vi "Read Waveform Measurement.vi"(6 "Source 2 (21: None)":u16(ring)=21 items=["Channel 1", "Channel 2", "Channel 3", "Channel 4", "DIG 0", "DIG 1", "DIG 2", "DIG 3", "DIG 4", "DIG 5", "DIG 6", "DIG 7", "DIG 8", "DIG 9", "DIG 10", "DIG 11", "DIG 12", "DIG 13", "DIG 14", "DIG 15", "Math", "None"], 8 "error in (no error)":errorcluster, 9 "Measurement Function (7: Frequency)":u16(ring)=7 items=["Amplitude", "Voltage Average", "Base", "Counter", "Delay", "Duty Cycle", "Fall Time", "Frequency", "Voltage Max", "Voltage Min", "Overshoot", "Voltage Vpp", "Period", "Phase", "Preshoot", "Rise Time", "Voltage RMS", "Top", "Width Positive", "X at Max Y", "X at Min Y"], 10 "Source 1 (0: Channel 1)":u16(ring) items=["Channel 1", "Channel 2", "Channel 3", "Channel 4", "DIG 0", "DIG 1", "DIG 2", "DIG 3", "DIG 4", "DIG 5", "DIG 6", "DIG 7", "DIG 8", "DIG 9", "DIG 10", "DIG 11", "DIG 12", "DIG 13", "DIG 14", "DIG 15", "Math"], 11 "VISA resource name":refnum<visa-resource-name>="GPIB0::1::INSTR") -> (0 "error out":errorcluster, 2 "Measured Value":dbl, 3 "VISA resource name out":refnum<visa-resource-name>)   [LabVIEW 2021, in "Agilent 6000 Series.lvlib"]
doc: "This VI initiates an acquisition on the channels that you enable with the ag6000a Configure Channel.vi. It then waits for the acquisition to complete, obtains a waveform measurement on the channel you specify, and returns the measurement value. You specify a particular measurement type, such as rise time, frequency, and voltage peak-to-peak. You can call the ag6000a Fetch Waveform Measurement.vi separately for any other waveform measurement that you want to obtain on a specific channel without initiating another acquisition.\n\nNotes:\n(1) You must configure the appropriate reference levels before you call this VI to take a rise time, fall time, width negative, width positive, duty cycle negative, or duty cycle positive measurement.\n(2) You configure the low, mid, and high references either by calling the ag6000a Configure Reference Levels.vi."
uses:
  Agilent 6000 Series.lvlib
  Low Data VIs/Fetch Waveform Measurement.vi
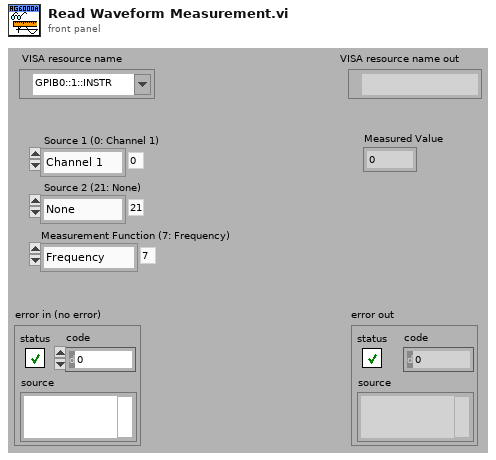
[diagram p1: front panel]
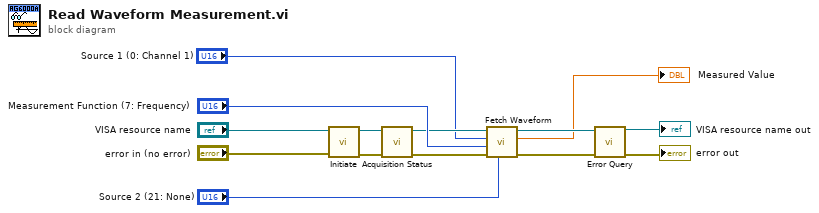
[diagram p0: block diagram]
diagram:
  n1 = call "Initiate.vi"("error in (no error)"="error in (no error)", "VISA resource name"="VISA resource name") -> ("error out"=w6:errorcluster, "VISA resource name out"=w5:refnum<visa-resource-name>)  [unwired: 8 in]
  n2 = call "Acquisition Status.vi"("error in (no error)"=w6, "VISA resource name"=w5) -> ("error out"=w3:errorcluster, "VISA resource name out"=w4:refnum<visa-resource-name>)  [unwired: 7 in, 1 out]
  n3 = call-poly "Fetch Waveform.vi"("Source 2 (21: None)"="Source 2 (21: None)", "error in (no error)"=w3, "Measurement Function (7: Frequency)"="Measurement Function (7: Frequency)", "Source 1 (0: Channel 1)"="Source 1 (0: Channel 1)", "VISA resource name"=w4) -> ("error out"=w9:errorcluster, "Measured Value"=→"Measured Value":dbl, "VISA resource name out"=w10:refnum<visa-resource-name>)  [unwired: 4 in]
  n4 = call "Error Query.vi"("error in (no error)"=w9, "VISA resource name"=w10) -> ("error out"=→"error out":errorcluster, "VISA resource name out"=→"VISA resource name out":refnum<visa-resource-name>)  [unwired: 6 in, 2 out]
